vi "unique_history.vi"(10 "History In":cluster{"Time Stamp":timestamp, "Path":path}[](array[cluster])) -> (0 "uFiles":path[](array[path]), 2 "History Out":cluster{"Time Stamp":timestamp, "Path":path}[](array[cluster]))   [LabVIEW 2015, in "oskar_tools.lvlib"]
uses:
  oskar_tools.lvlib
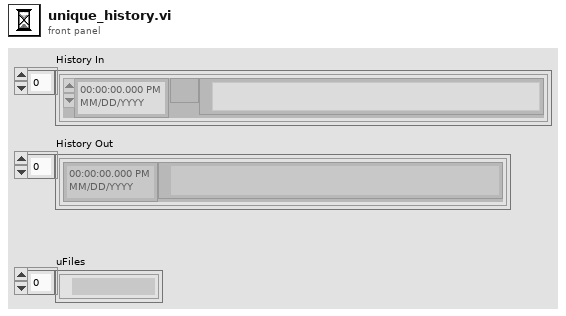
[diagram p1: front panel]
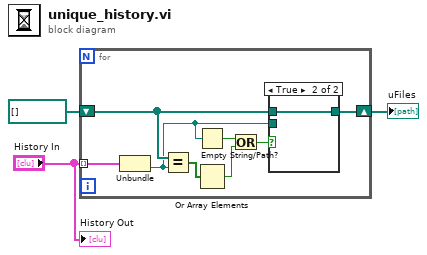
[diagram p0: block diagram]
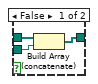
[diagram p2: hidden frame]
diagram:
  n1 = for {
    tunnel: "History In" -> [w11] mode=indexing
    shift-right: [w10] -> w1
    shift-left: path[] [] ("Array") -> [w9]
    n2 = Unbundle(w11) -> ("Path"=w4:path)  [unwired: 1 out]
    n3 = Equal?(x=w9, y=w4) -> (x = y?=w8:bool[])
    n4 = Empty String/Path?(string/path=w4) -> (empty?=w5:bool)
    n5 = Or Array Elements(Boolean array=w8) -> (logical OR=w7:bool)
    n6 = Or(x=w5, y=w7) -> (x .or. y?=w6:bool)
    n7 = case shown="True" w6 {
      tunnel: w4 -> [w14 _]
      tunnel: w9 -> [w13 w15]
      tunnel: [w12 w15] -> w10
      frame False {
        n8 = Build Array (concatenate)(w13, w14) -> (w12:path[])
      }
      frame True {
      }
    }
  }
  "uFiles" <- w1
  "History Out" <- "History In"
